vi "write serial number.vi"(8 "error in":errorcluster, 10 "serial number":string, 11 "device in":refnum<class "Device.lvclass">) -> (0 "error out":errorcluster, 3 "device out":refnum<class "Device.lvclass">)   [LabVIEW 2013, in "SMI.lvlib" / "Device.lvclass"]
uses:
  Device.lvclass
  Device.lvclass/Device.ctl
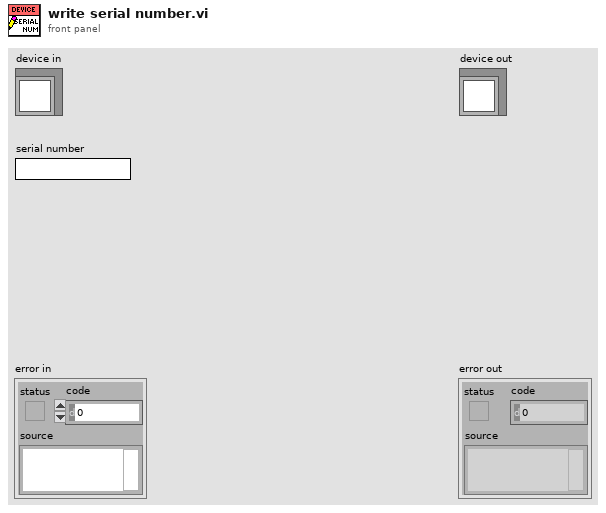
[diagram p1: front panel]
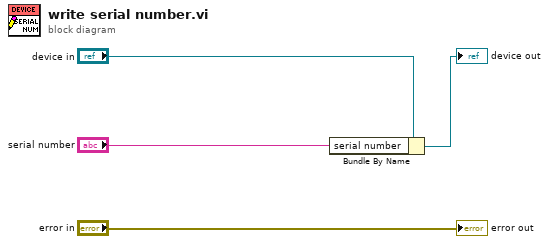
[diagram p0: block diagram]
diagram:
  n1 = Bundle By Name(cluster="device in", "serial number"="serial number") -> (→"device out":refnum<class "Device.lvclass">)
  "error out" <- "error in"
